vi "Copy_Paste.vi"() -> ()   [LabVIEW 2021]
panel:
  in  "Local Folder Location":path
  in  "Source File Location":path
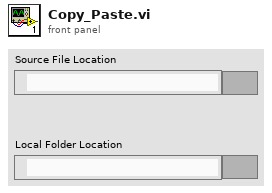
[diagram p1: front panel]
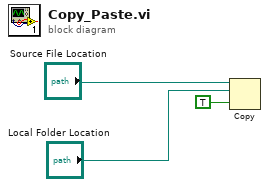
[diagram p0: block diagram]
diagram:
  n1 = Copy(9:TRUE ("overwrite (F)"), 10:"Local Folder Location", 11:"Source File Location") -> ()  [unwired: 2 in, 3 out]
